vi "VFH Choose Heading.vi"(0 "histogram in":dbl[](array[numeric]), 2 "inner visibility threshold":dbl, 3 "outer visibility threshold":dbl, 5 "last commanded heading (rad)":dbl, 7 "current heading (rad)":dbl, 9 "target heading (rad)":dbl, 11 "mask in":bool[](array[boolean]), 13 "maximum heading change (rad)":dbl=1.57) -> (6 "chosen heading (rad)":dbl, 8 "heading found?":bool, 15 "mask out":bool[](array[boolean]))   [LabVIEW 2017, in "NI_Robotics_Vector Field Histogram.lvlib"]
uses:
  <vilib>/robotics/Obstacle Avoidance/Advanced Vector Field Histogram/NI_Robotics_Vector Field Histogram.lvlib
  <vilib>/Analysis/coordinate.llb/Wrap Angle (scalar).vi
  <vilib>/Analysis/NI_AAL_Angle.lvlib
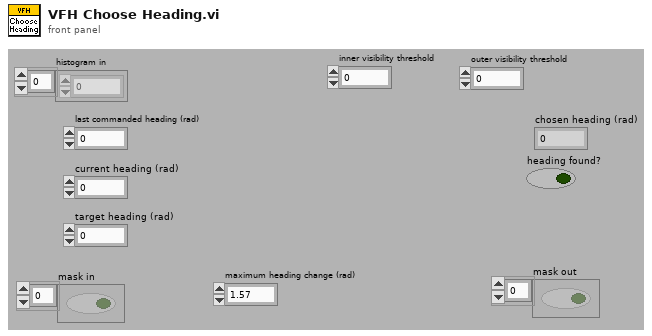
[diagram p1: front panel]
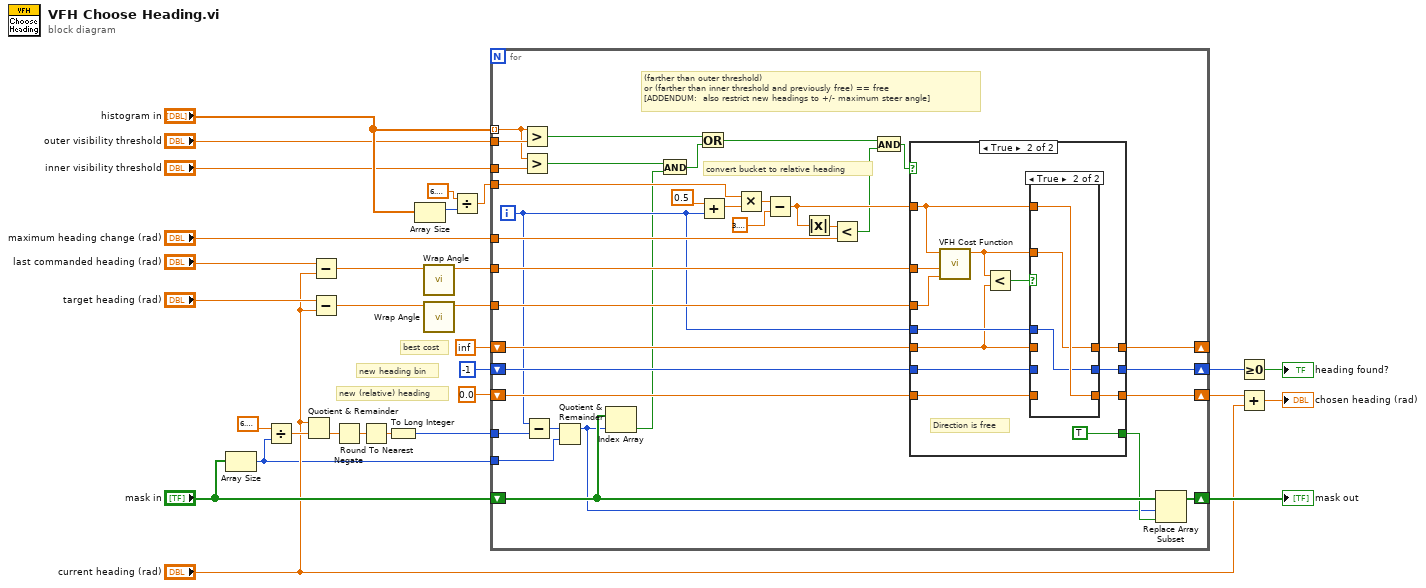
[diagram p0: block diagram]
diagram:
  # "best cost"
  # "new heading bin"
  # "new (relative) heading"
  n1 = Array Size(array="mask in") -> (size(s)=w5:i32)
  n2 = Divide(x=6.283185307179586, y=w5) -> (x/y=w17:dbl)
  n3 = Quotient & Remainder(x="current heading (rad)", y=w17) -> (floor(x/y)=w18:dbl)  [unwired: 1 out]
  n4 = Subtract(x="last commanded heading (rad)", y="current heading (rad)") -> (x-y=w4:dbl)
  n5 = Subtract(x="target heading (rad)", y="current heading (rad)") -> (x-y=w2:dbl)
  n6 = Negate(x=w18) -> (-x=w19:dbl)
  n7 = Round To Nearest(number=w19) -> (nearest integer value=w20:dbl)
  n8 = To Long Integer(number=w20) -> (32bit integer=w30:i32)
  n9 = Array Size(array="histogram in") -> (size(s)=w24:i32)
  n10 = call-poly <vilib>:"Wrap Angle.vi"("angle in"=w4) -> ("angle out"=w3:dbl)  [unwired: 9 in, 1 out]
  n11 = call-poly <vilib>:"Wrap Angle.vi"("angle in"=w2) -> ("angle out"=w1:dbl)  [unwired: 9 in, 1 out]
  n12 = Divide(x=6.283185307179586, y=w24) -> (x/y=w27:dbl)
  n13 = for {
    tunnel: "histogram in" -> [w40] mode=indexing
    shift-right: [w59] -> w14
    shift-left: -1 -> [w61]
    tunnel: "outer visibility threshold" -> [w64]
    shift-right: [w60] -> _
    shift-left: inf -> [w62]
    tunnel: w27 -> [w63]
    tunnel: w1 -> [w58]
    shift-right: [w56] -> w23
    shift-left: 0.0 -> [w57]
    tunnel: "inner visibility threshold" -> [w55]
    tunnel: "maximum heading change (rad)" -> [w45]
    tunnel: w3 -> [w41]
    tunnel: w30 -> [w38]
    tunnel: w5 -> [w36]
    shift-right: [w31] -> w28
    shift-left: "mask in" -> [w34]
    i -> [w39]
    # "convert bucket to relative heading"
    # "(farther than outer threshold) \nor (farther than inner threshold and previously free) == free\n[ADDENDUM:  also restrict new headings to +/- maximum steer angle]"
    n14 = Greater?(x=w40, y=w64) -> (0:w54:bool)
    n15 = Greater?(x=w40, y=w55) -> (0:w53:bool)
    n16 = Subtract(x=w39, y=w38) -> (x-y=w37:i32)
    n17 = Quotient & Remainder(x=w37, y=w36) -> (x-y*floor(x/y)=w32:i32)  [unwired: 1 out]
    n18 = Index Array(array=w34, index=w32) -> (element=w35:bool)
    n19 = And(x=w53, y=w35) -> (x .and. y?=w52:bool)
    n20 = Or(x=w54, y=w52) -> (x .or. y?=w43:bool)
    n21 = Add(x=0.5, y=w39) -> (x+y=w50:dbl)
    n22 = Multiply(x=w63, y=w50) -> (x*y=w49:dbl)
    n23 = Subtract(x=w49, y=3.141592653589793) -> (x-y=w47:dbl)
    n24 = Absolute Value(x=w47) -> (abs(x)=w46:dbl)
    n25 = Less?(x=w46, y=w45) -> (x < y?=w44:bool)
    n26 = And(x=w43, y=w44) -> (x .and. y?=w42:bool)
    n27 = case shown="True" w42 {
      tunnel: w39 -> [_ w80]
      tunnel: w62 -> [w67 w79]
      tunnel: w61 -> [w66 w78]
      tunnel: [w67 w77] -> w60
      tunnel: [w66 w76] -> w59
      tunnel: w58 -> [_ w75]
      tunnel: w57 -> [w65 w74]
      tunnel: [w65 w73] -> w56
      tunnel: [_ TRUE] -> w33
      tunnel: w47 -> [_ w68]
      tunnel: w41 -> [_ w69]
      frame False {
        # "Direction is Blocked"
      }
      frame True {
        # "Direction is free"
        n28 = call <vilib>:"VFH Cost Function.vi"("target heading (relative to current)"=w75, "last commanded heading (relative to current)"=w69, "candidate heading (relative to current)"=w68) -> ("cost"=w70:dbl)  [unwired: 8 in]
        n29 = Less?(x=w70, y=w79) -> (x < y?=w71:bool)
        n30 = case shown="True" w71 {
          tunnel: w68 -> [_ w86]
          tunnel: w70 -> [_ w85]
          tunnel: w79 -> [w83 _]
          tunnel: w78 -> [w82 _]
          tunnel: w74 -> [w81 _]
          tunnel: [w81 w86] -> w73
          tunnel: [w83 w85] -> w77
          tunnel: w80 -> [_ w84]
          tunnel: [w82 w84] -> w76
          frame False {
          }
          frame True {
          }
        }
      }
    }
    n31 = Replace Array Subset(array=w34, new element=w33, index=w32) -> (w31:bool[])
  }
  "mask out" <- w28
  n32 = Greater Or Equal To 0?(x=w14) -> (x >= 0?=→"heading found?":bool)
  n33 = Add(x=w23, y="current heading (rad)") -> (x+y=→"chosen heading (rad)":dbl)
